vi "Receiver.vi"() -> ()   [LabVIEW 2016]
uses:
  Global Variable.vi
panel:
  out "Random Data Reading":dbl(graph)
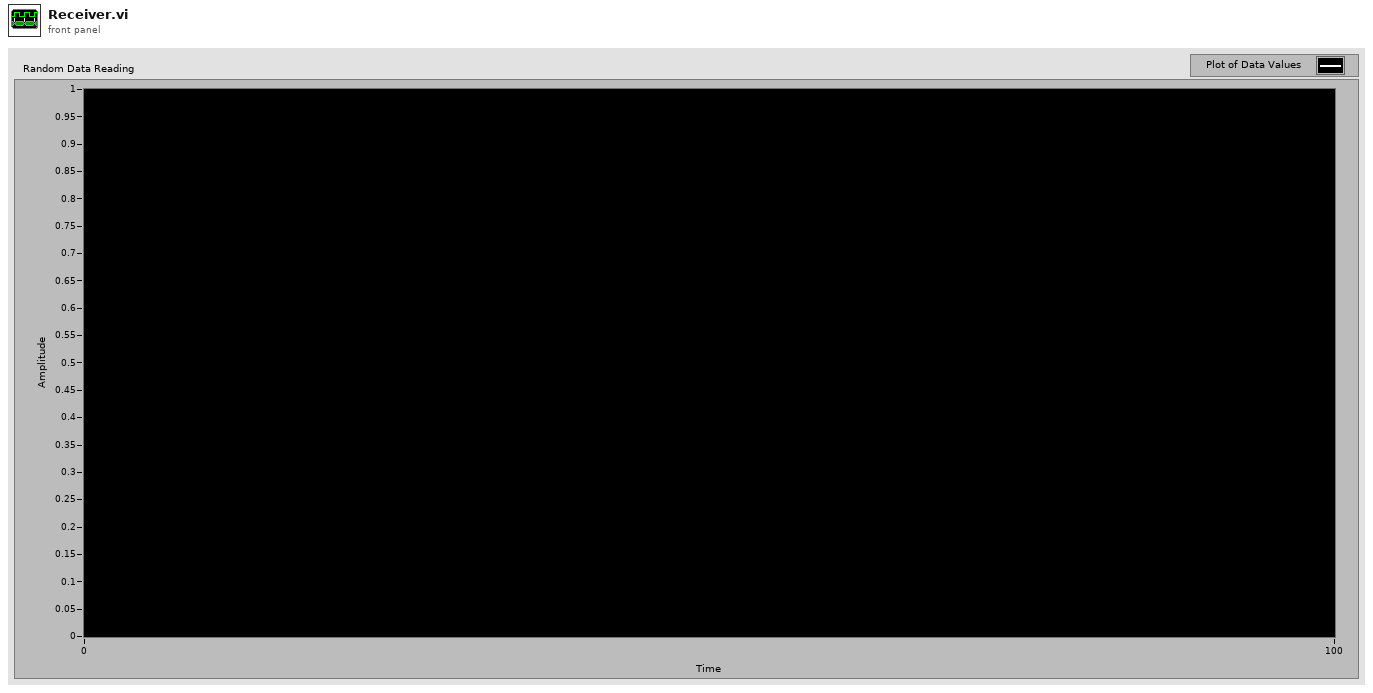
[diagram p1: front panel]
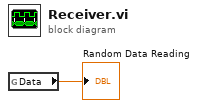
[diagram p0: block diagram]
diagram:
  n1 = global read "Global Variable.vi" "Data"() -> (→"Random Data Reading":dbl)
